vi "Set Transfer Group Timeout Behavior.vi"(8 "error in (no error)":errorcluster, 10 "timeout behavior":T1, 11 "transfer group in":T2={"core"={"name"="Group", "direction"=enum."Rx", "cycle timing"={"priority"=0, "decimation"=0, "offset"=255}, "timeout behavior"=enum."Throw Error"}, "component settings"=[], "transfers"=[]} {"transfers"."channels"."core"."string offset" format="%d bytes"}) -> (0 "error out":errorcluster, 3 "transfer group out":T2={"core"={"name"="Group", "direction"=enum."Rx", "cycle timing"={"priority"=0, "decimation"=0, "offset"=255}, "timeout behavior"=enum."Throw Error"}, "component settings"=[], "transfers"=[]} {"transfers"."channels"."core"."string offset" format="%d bytes"})   [LabVIEW 2017, in "DSF Core.lvlib" / "Configuration Session.lvclass"]
uses:
  Configuration Session.lvclass
  Typedefs/DSF Engine Transfer Group Configuration.ctl
  Typedefs/DSF Core Group Configuration.ctl
  Typedefs/DSF Direction.ctl
  Typedefs/DSF Timing Info.ctl
  Typedefs/DSF Timeout Behavior.ctl
  Typedefs/DSF Settings Info.ctl
  Typedefs/DSF Version Info.ctl
  Typedefs/DSF Engine Transfer Configuration.ctl
  Typedefs/DSF Core Transfer Configuration.ctl
  Typedefs/DSF Engine Channel Configuration.ctl
  Typedefs/DSF Core Channel Configuration.ctl
  Typedefs/DSF Data Type.ctl
  DSF Core.lvlib
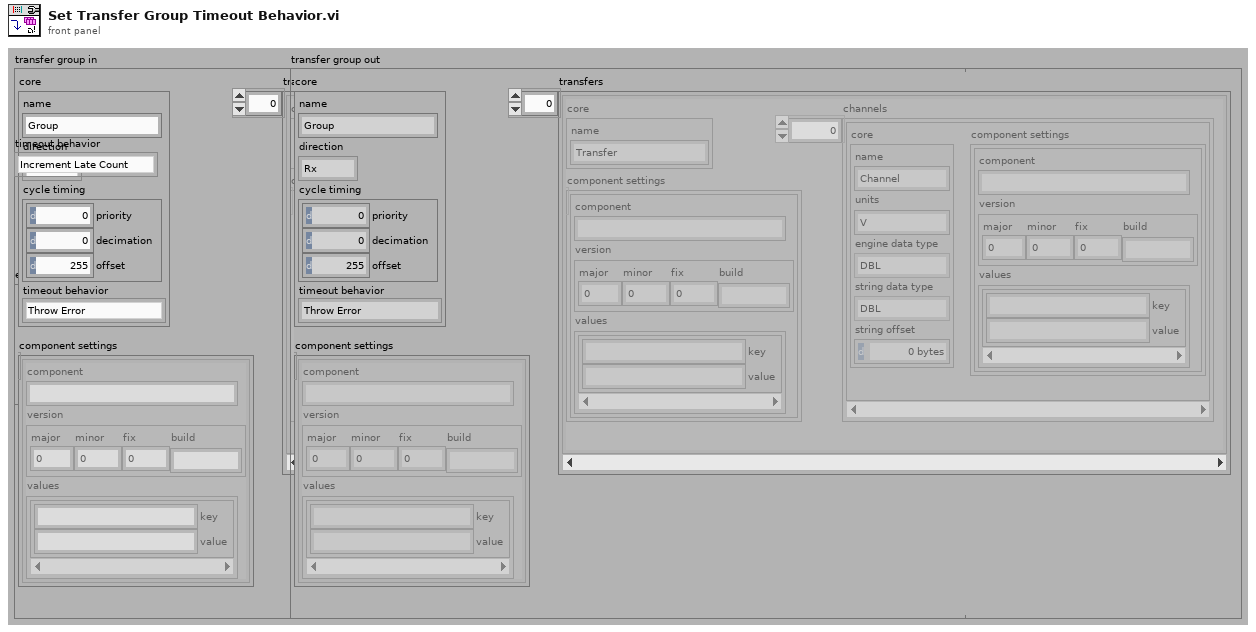
[diagram p1: front panel]
types:
  T1 = typedef "DSF Core.lvlib/DSF Timeout Behavior.ctl" = enum8{"Increment Late Count", "Throw Error"}
  T2 = typedef "DSF Core.lvlib/DSF Engine Transfer Group Configuration.ctl" = cluster{"core":T3, "component settings":T6[], "transfers":T8[]}
  T3 = typedef "DSF Core.lvlib/DSF Core Group Configuration.ctl" = cluster{"name":string, "direction":T4, "cycle timing":T5, "timeout behavior":T1}
  T4 = typedef "DSF Core.lvlib/DSF Direction.ctl" = enum8{"Tx", "Rx"}
  T5 = typedef "DSF Core.lvlib/DSF Timing Info.ctl" = cluster{"priority":u64, "decimation":u64, "offset":u64}
  T6 = typedef "DSF Core.lvlib/DSF Settings Info.ctl" = cluster{"component":string, "version":T7, "values":cluster{"key":string, "value":string}[]}
  T7 = typedef "DSF Core.lvlib/DSF Version Info.ctl" = cluster{"major":u32, "minor":u32, "fix":u32, "build":string}
  T8 = typedef "DSF Core.lvlib/DSF Engine Transfer Configuration.ctl" = cluster{"core":T9, "component settings":T6[], "channels":T10[]}
  T9 = typedef "DSF Core.lvlib/DSF Core Transfer Configuration.ctl" = cluster{"name":string}
  T10 = typedef "DSF Core.lvlib/DSF Engine Channel Configuration.ctl" = cluster{"core":T11, "component settings":T6[]}
  T11 = typedef "DSF Core.lvlib/DSF Core Channel Configuration.ctl" = cluster{"name":string, "units":string, "engine data type":T12, "string data type":T12, "string offset":u64}
  T12 = typedef "DSF Core.lvlib/DSF Data Type.ctl" = enum8{"Bool", "SGL", "DBL", "I8", "I16", "I32", "I64", "U8", "U16", "U32", "U64"}
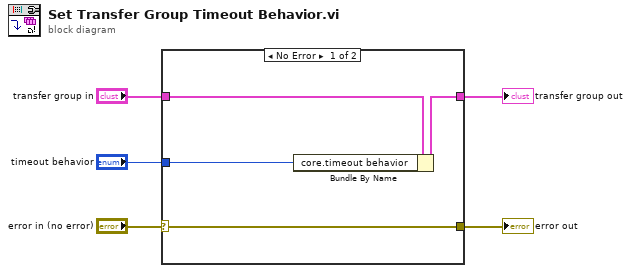
[diagram p0: block diagram]
diagram:
  n1 = case shown="No Error" "error in (no error)" {
    selector: "error in (no error)" -> [w7 w11]
    tunnel: [w7 w11] -> w5
    tunnel: [w8 w10] -> w2
    tunnel: "transfer group in" -> [w9 w10]
    tunnel: "timeout behavior" -> [w6 _]
    frame No Error {
      n2 = Bundle By Name(cluster=w9, "core.timeout behavior"=w6) -> (w8:T2)
    }
    frame Error {
    }
  }
  "error out" <- w5
  "transfer group out" <- w2
